vi "Kpro Read String Pot 2016.vi"(0 "Read String Pot":bool, 1 "Feet of\nStainless to be\nUsed (Count) in":i32, 2 "Session Array in":dbl[][](array[numeric]), 3 "Flow":dbl, 4 "Manual Depth In":dbl, 5 "Finished In":bool, 6 "Depth Cluster in":T1, 7 "error in (no error)":errorcluster, 8 "String Pot \nSlope in":dbl=1.7339999675750732 format="%.2f", 9 "Sensor Cluster In in":T2, 10 "Descriptions":string[](array[string]), 11 "Pressure in":dbl format="%.2f", 12 "Array in":refnum<k24>[](array[refnum]), 13 "Downhole Pressure Sensor":dbl format="%#_13g") -> (18 "Sensor Cluster 2":T2, 19 "IK":dbl, 20 "Array out":refnum<k24>[](array[refnum]), 21 "Generate Array Calc IK":bool, 22 "Finish Take Data":bool, 23 "Depth Rate":dbl format="%.2f", 24 "Feet of\nStainless to be\nUsed (Count) out":i32, 25 "Depth Cluster out":T1, 26 "Single String Pot Session Array out":dbl[][](array[numeric]))   [LabVIEW 2016]
uses:
  Waterloo DAQ/controls/MCC DAQ Readings.ctl
  C:/Program Files (x86)/National Instruments/LabVIEW 2016/vi.lib/ULx/ULx_LV.dll
  Waterloo DAQ/controls/Kpro hydraulic measurement cluster.ctl
panel:
  out "x .or. y?":bool
  out "Filter Output":dbl
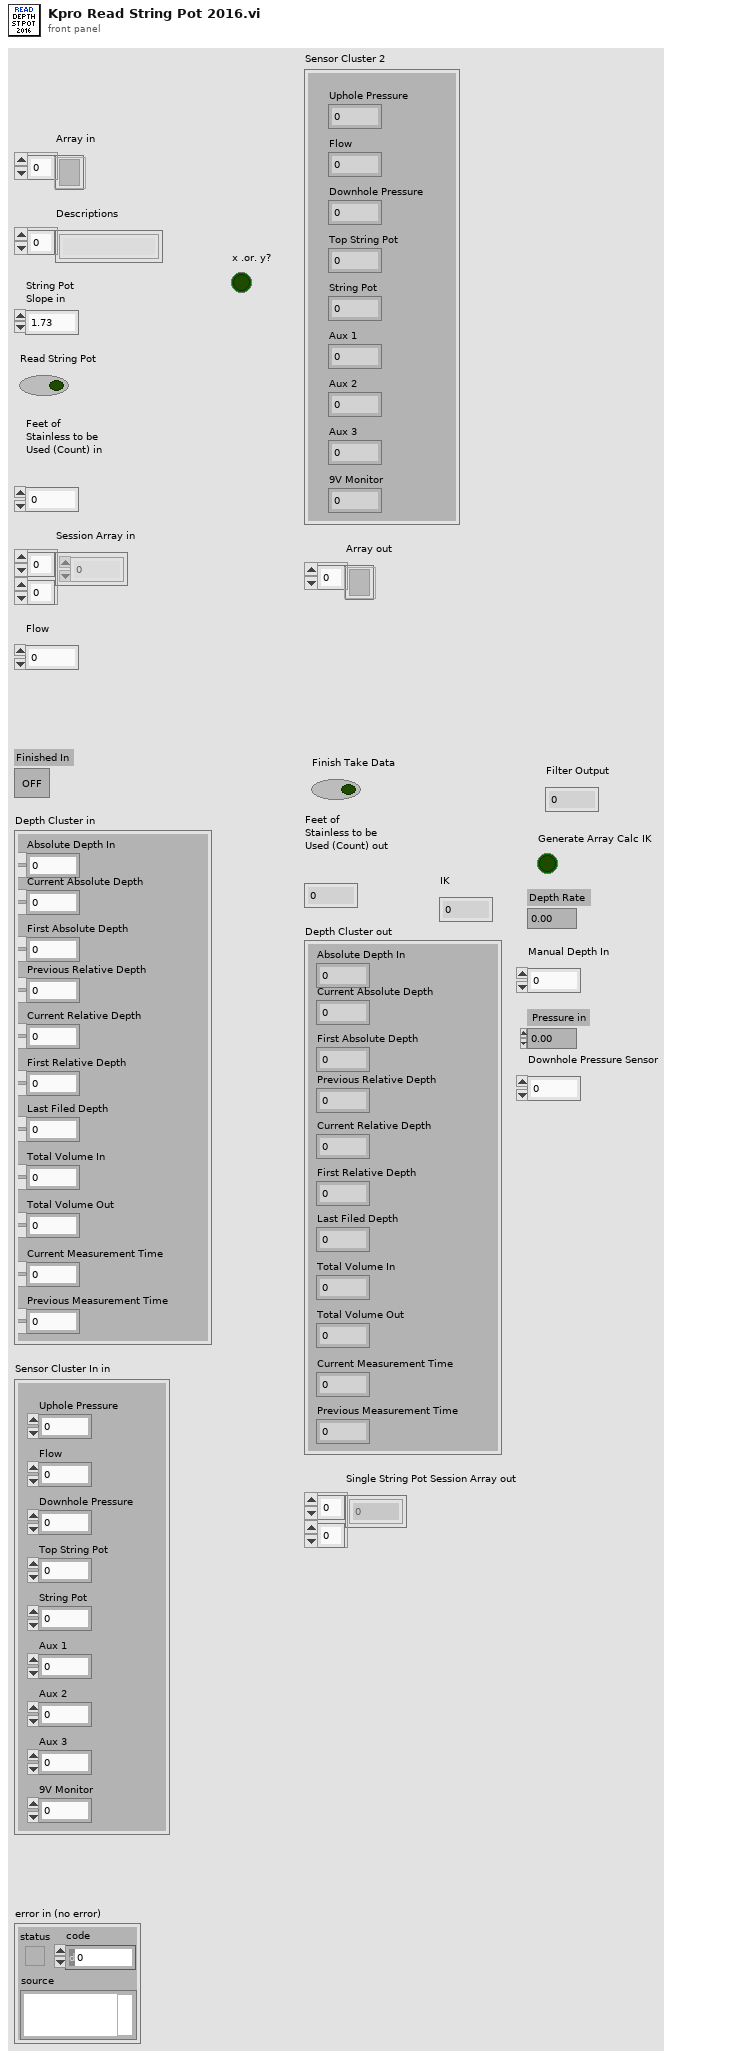
[diagram p1: front panel]
types:
  T1 = typedef "Kpro hydraulic measurement cluster.ctl" = cluster{"Absolute Depth In":dbl, "Current Absolute Depth":dbl, "First Absolute Depth":dbl, "Previous Relative Depth":dbl, "Current Relative Depth":dbl, "First Relative Depth":dbl, "Last Filed Depth":dbl, "Total Volume In":dbl, "Total Volume Out":dbl, "Current Measurement Time":dbl, "Previous Measurement Time":dbl}
  T2 = typedef "MCC DAQ Readings.ctl" = cluster{"Uphole Pressure":dbl, "Flow":dbl, "Downhole Pressure":dbl, "Top String Pot":dbl, "String Pot":dbl, "Aux 1":dbl, "Aux 2":dbl, "Aux 3":dbl, "9V Monitor":dbl}
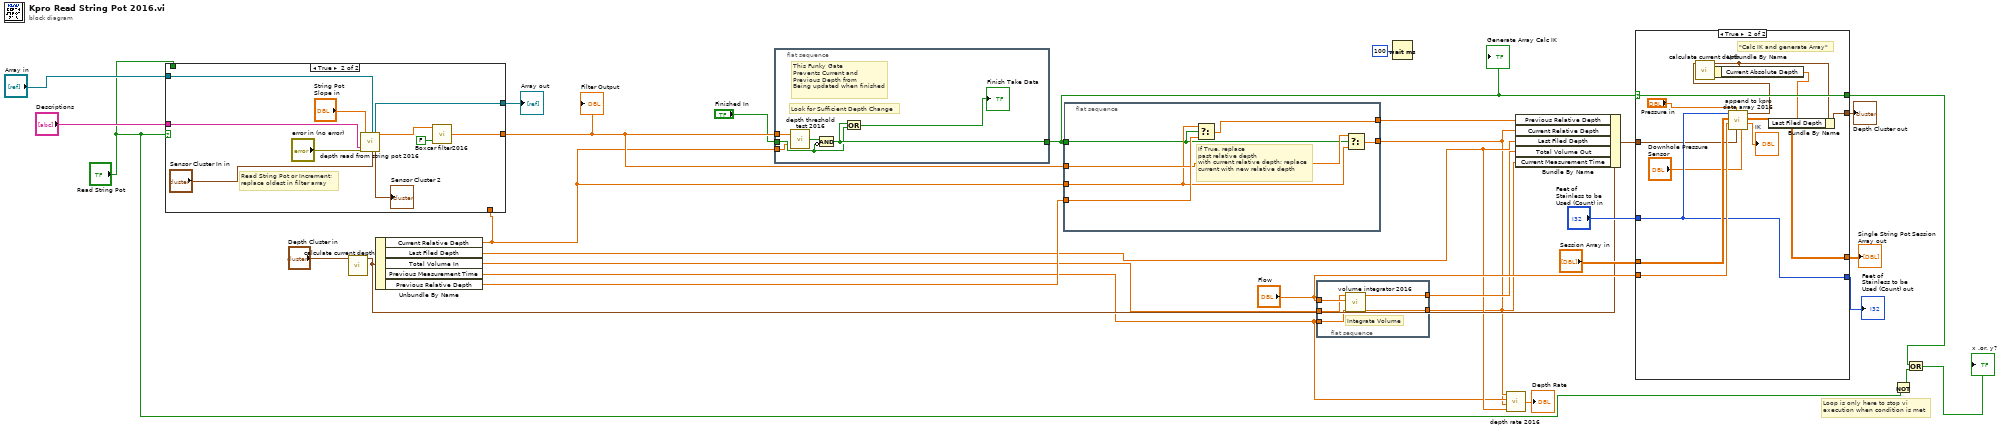
[diagram p0: block diagram]
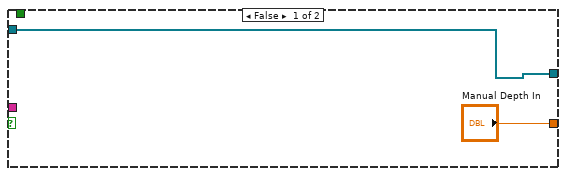
[diagram p2: hidden frame]
diagram:
  # "Loop is only here to stop vi \nexecution when condition is met"
  n1 = call "calculate current depth.vi"("Cluster in"="Depth Cluster in") -> ("Cluster out"=w20:T1)  [unwired: 10 in]
  n2 = Unbundle By Name(w20) -> ("Current Relative Depth"=w7:dbl, "Last Filed Depth"=w10:dbl, "Total Volume In"=w15:dbl, "Previous Measurement Time"=w8:dbl, "Previous Relative Depth"=w18:dbl)
  n3 = case shown="True" "Read String Pot" {
    tunnel: ["Manual Depth In" w41] -> w14
    tunnel: "Read String Pot" -> [_ _]
    tunnel: "Descriptions" -> [_ w40]
    tunnel: [w32 w37] -> w29
    tunnel: "Array in" -> [w32 w36]
    tunnel: w7 -> [_ _]
    frame False {
    }
    frame True {
      # "Read String Pot or Increment;\nreplace oldest in filter array"
      n4 = call "depth read from string pot 2016.vi"("Descriptions"=w40, "error in (no error)"="error in (no error)", "String Pot \nSlope"="String Pot \nSlope in", "Array in"=w36, "Sensor Cluster In"="Sensor Cluster In in") -> ("Array out"=w37:refnum<k24>[], "Sensor Cluster 2"=→"Sensor Cluster 2":T2, "Depth"=w42:dbl)  [unwired: 11 in, 1 out]
      n5 = call "Boxcar filter2016.vi"("Initialize"=FALSE, "Filter Input"=w42) -> ("Filter Output"=w41:dbl)  [unwired: 1 in]
    }
  }
  "Array out" <- w29
  "Filter Output" <- w14
  n6 = flat-sequence {
    tunnel: [w47] -> w12
    tunnel: "Finished In" -> [w46]
    tunnel: w14 -> [w45]
    tunnel: w7 -> [w44]
    frame #0 {
      # "Look for Sufficient Depth Change"
      # "This Funky Gate\nPrevents Current and \nPrevious Depth from \nBeing updated when finished"
      n7 = call "depth threshold test 2016.vi"("Depth\nPrevious"=w44, "Depth \nCurrent"=w45) -> ("Threshold\nExceeded"=w48:bool)
      n8 = Compound Arithmetic op=AND(w48, invert w46) -> (w47:bool)
      n9 = Or(x=w47, y=w46) -> (x .or. y?=→"Finish Take Data":bool)
    }
  }
  n10 = flat-sequence {
    tunnel: [w54] -> w17
    tunnel: w18 -> [w53]
    tunnel: [w52] -> w1
    tunnel: w12 -> [w49]
    tunnel: w14 -> [w51]
    tunnel: w7 -> [w50]
    frame #0 {
      # "If True, replace\npast relative depth\nwith current relative depth; replace\ncurrent with new relative depth"
      n11 = Select(t=w50, s=w49, f=w53) -> (s? t:f=w54:dbl)
      n12 = Select(t=w51, s=w49, f=w50) -> (s? t:f=w52:dbl)
    }
  }
  n13 = flat-sequence {
    tunnel: w8 -> [w59]
    tunnel: [w58] -> w9
    tunnel: "Flow" -> [w57]
    tunnel: w15 -> [w56]
    tunnel: [w55] -> w16
    frame #0 {
      # "Integrate Volume"
      n14 = call "volume integrator 2016.vi"("Previous Time (sec)"=w59, "Flow"=w57, "Total Volume in"=w56) -> ("Current Time (sec)"=w58:dbl, "Total Volume Out mL"=w55:dbl)  [unwired: 3 in]
    }
  }
  n15 = Wait (ms)(milliseconds to wait=u32 100) -> ()  [unwired: 1 out]
  n16 = call "depth rate 2016.vi"("Depth Last"=w10, "Depth Current"=w1, "Time Last"=w8, "Time Current"=w9) -> ("Depth Rate"=→"Depth Rate":dbl)
  n17 = Bundle By Name(cluster=w20, "Previous Relative Depth"=w17, "Current Relative Depth"=w1, "Last Filed Depth"=w10, "Total Volume Out"=w16, "Current Measurement Time"=w9) -> (w21:T1)
  n18 = case shown="True" w12 {
    selector: w12 -> [w61 w69]
    tunnel: "Session Array in" -> [w60 w76]
    tunnel: [w60 w75] -> w24
    tunnel: "Feet of\nStainless to be\nUsed (Count) in" -> [w62 w72]
    tunnel: "Flow" -> [_ w74]
    tunnel: [w63 w68] -> w22
    tunnel: w21 -> [w63 w67]
    tunnel: [w62 w72] -> w27
    tunnel: [w61 w69] -> w6
    frame False {
    }
    frame True {
      # "\"Calc IK and generate Array\""
      n19 = call "append to kpro data array 2016.vi"("Downhole Pressure Sensor"="Downhole Pressure Sensor", "Cluster in"=w67, "Up hole Pressure Sensor"="Pressure in", "Flow"=w74, "Corrected Array in"=w76, "Feet of\nStainless to be\nUsed (Count) in"=w72) -> ("IK"=→"IK":dbl, "Array Out"=w75:dbl[][], "Cluster out 2"=w66:T1)  [unwired: 2 in, 1 out]
      n20 = call "calculate current depth.vi"("Cluster in"=w66) -> ("Cluster out"=w65:T1)  [unwired: 10 in]
      n21 = Unbundle By Name(w65) -> ("Current Absolute Depth"=w64:dbl)
      n22 = Bundle By Name(cluster=w65, "Last Filed Depth"=w64) -> (w68:T1)
    }
  }
  "Feet of\nStainless to be\nUsed (Count) out" <- w27
  "Single String Pot Session Array out" <- w24
  "Depth Cluster out" <- w22
  n23 = Not(x="Read String Pot") -> (.not. x?=w2:bool)
  n24 = Or(x=w6, y=w2) -> (x .or. y?=→"x .or. y?":bool)
  "Generate Array Calc IK" <- w12
